vi "DSA AI and AO.vi"() -> ()   [LabVIEW 2014]
doc: "Overview:\nThis VI demonstrates generation and acquisition of a broadband signal to perform measurement of the frequency response of your device.\n\nRequirements:\nLabVIEW Full Development System\nSound and Vibration Toolkit\n\nInstructions:\n1. Connect DUT to DAQmx hardware.\n2. Specify connected output channel and input channel.\n3. Use SVL Measure Propagation Delay (DAQmx) VI to measure device propagation delay [samples].\n4. Run the VI.\n\nDetails:\nThis VI generates and acquires data for an averaged frequency response measurement. This VI performs a continuous acquisition and stops when the averaged measurement is complete. You specify the sampling frequency, block size, and averaging parameters to use for the frequency response measurement. \n\nThe graph outputs display the acquired stimulus and response signals versus time and the magnitude and phase of the frequency response versus frequency."
uses:
  <vilib>/addons/_NISVFA/_Shared subVIs/Controls/svc_Window.ctl
  <vilib>/Utility/error.llb/DialogType.ctl
  <vilib>/DAQmx/create/channels.llb/DAQmx Create Channel (AI-Voltage-Basic).vi
  <vilib>/DAQmx/configure/timing.llb/DAQmx Timing (Sample Clock).vi
  <vilib>/DAQmx/create/channels.llb/DAQmx Create Channel (AO-Voltage-Basic).vi
  <vilib>/DAQmx/configure/trigger.llb/DAQmx Start Trigger (Digital Edge).vi
  <vilib>/DAQmx/write.llb/DAQmx Write (Analog 2D DBL NChan NSamp).vi
  <vilib>/DAQmx/read.llb/DAQmx Read (Analog 1D Wfm NChan NSamp).vi
  <vilib>/addons/_NISVFA/_Baseband FFT/SVFA Power Spectrum (1 Ch).vi
  <vilib>/Analysis/NI_AALBase.lvlib
  <resource>/objmgr/daqmx.rc
  <vilib>/measure/NI_MABase.lvlib
panel:
  out "DC 2":dbl min=0.0 max=1.0 step=0.001 format="%.3f"
  out "DC 1":dbl min=0.0 max=1.0 step=0.001 format="%.3f"
  out "RMS 2":dbl min=0.0 max=1.0 step=0.001 format="%.3f"
  out "RMS 1":dbl min=0.0 max=1.0 step=0.001 format="%.3f"
  in  "stop":bool
  in  "Tab Control":enum32{"Time Record", "Power Spectum"}(tab)
  out "time record 2":waveform(dbl)[](graph)
  in  "sampling rate [Hz]":dbl=51200.0 format="%.2f"
  out "actual update rate":dbl=51200.0 format="%.2f"
  in  "excitation":T1(ring)=enum."Sine"
  in  "output physical channel":tag="PXI2Slot4/ao0:1"
  in  "input channel (stimulus)":tag="PXI2Slot4/ai0"
  in  "propagation delay [samples]":i32=1 min=1 step=1
  in  "amplitude":dbl=0.1 min=0.0 max=2.0 step=0.001 format="%.3f"
  in  "input channel (response)":tag="PXI2Slot4/ai1"
  in  "frequency":dbl=150.0 min=0.0 max=20000.0 step=0.1 format="%.1f"
  out "mag 2":cluster{"f0":dbl, "df":dbl, "magnitude":dbl[]}(graph)={"f0"=0.0, "df"=20.00000050524251, "magnitude"=[]}
  out "mag":cluster{"f0":dbl, "df":dbl, "magnitude":dbl[]}(graph)={"f0"=0.0, "df"=20.00000050524251, "magnitude"=[]}
  in  "block size":i32=16384 min=128
  in  "averaging parameters":T2={"averaging mode"=enum."RMS averaging", "weighting mode"=enum."Exponential", "number of averages"=10, "linear mode"=enum."One shot"} {"number of averages" min=1 step=1}
  in  "restart averaging":bool
  out "averages completed":dbl
  in  "window":T3=1 items=["None"=0, "Hanning"=1, "Hamming"=2, "Blackman-Harris"=3, "Exact Blackman"=4, "Blackman"=5, "Flat Top"=6, "4 Term B-Harris "=7, "7 Term B-Harris"=8, "Low Sidelobe"=9, "Force"=64, "Exponential"=65, "Blackman Nuttall"=11, "Triangle"=30, "Bartlett-Hanning"=31, "Bohman"=32, "Parzen"=33, "Welch"=34, "Kaiser"=60, "Dolph-Chebyshev"=61, "Gaussian"=62]
  in  "dB On":bool=TRUE
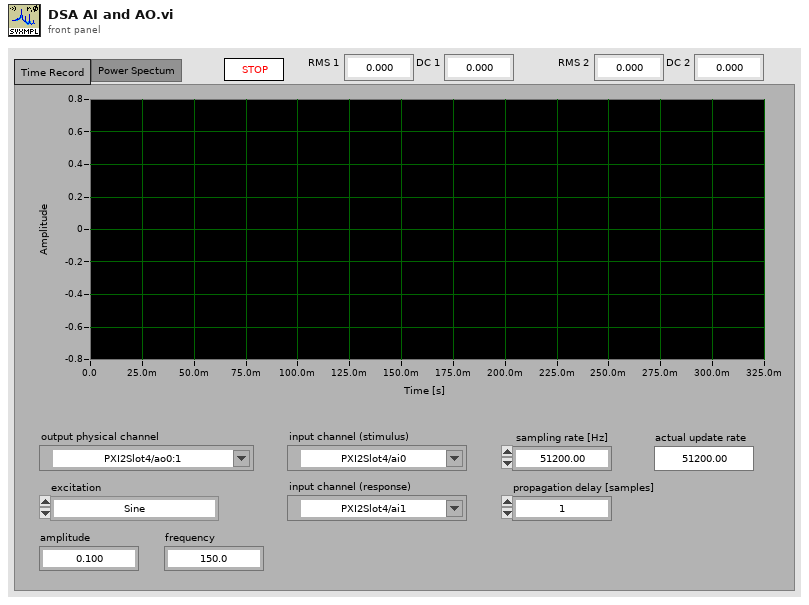
[diagram p1: front panel]
types:
  T1 = enum16{"uniform white noise", "Gaussian white noise", "periodic random noise", "Chirp", "Sine"}
  T2 = cluster{"averaging mode":enum16{"No averaging", "Vector averaging", "RMS averaging", "Peak hold"}, "weighting mode":enum16{"Linear", "Exponential"}, "number of averages":u32, "linear mode":enum16{"One shot", "Auto restart"}}
  T3 = typedef "svc_Window.ctl" = u32
  T4 = cluster{"coupling":i32, "enable IEPE excitation":bool, "IEPE current [mA]":dbl}
  T5 = typedef "DialogType.ctl" = u16
  T6 = cluster{"actual sample rate":dbl, "block size":i32}
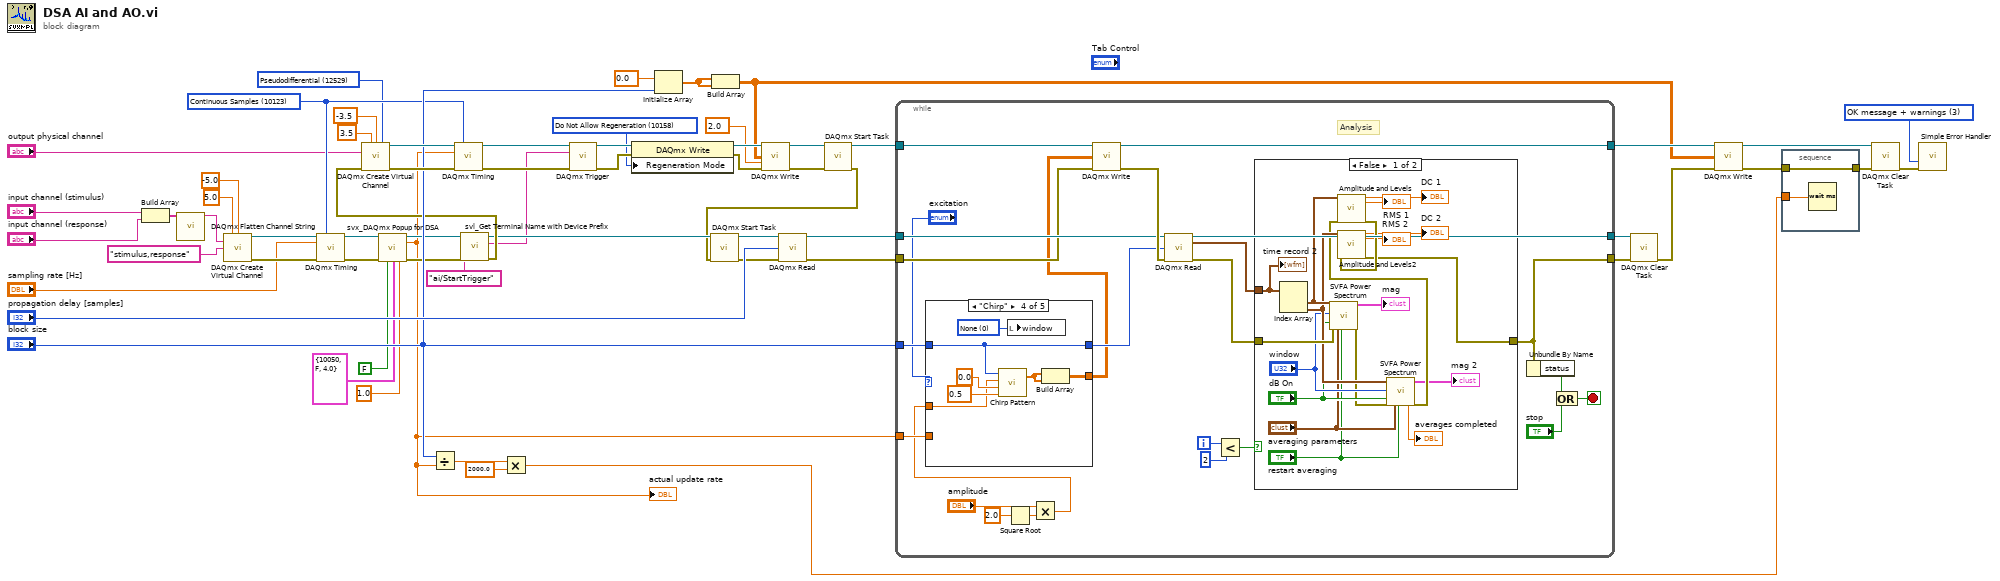
[diagram p0: block diagram]
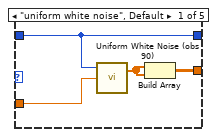
[diagram p2: hidden frame]
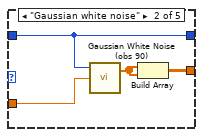
[diagram p3: hidden frame]
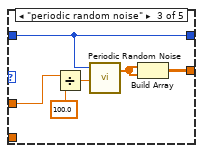
[diagram p4: hidden frame]
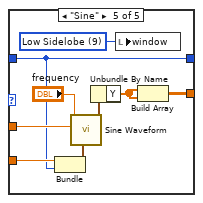
[diagram p5: hidden frame]
diagram:
  w3 = 12529 items=["Default"=-1, "RSE"=10083, "Differential"=10106, "Pseudodifferential"=12529] ("output terminal configuration")
  w30 = T5 3 items=["no dialog", "OK message", "continue or stop message", "OK message + warnings", "continue/stop + warnings"] ("type of dialog (OK msg:1)")
  w51 = 10158 items=["Allow Regeneration"=10097, "Do Not Allow Regeneration"=10158] ("RegenMode")
  w17 = 10123 items=["Finite Samples"=10178, "Continuous Samples"=10123] ("sample mode")
  n1 = Build Array("input channel (stimulus)", "input channel (response)") -> (w12:tag[])
  n2 = call <vilib>:"DAQmx Flatten Channel String.vi"("names in"=w12) -> ("names out"=w9:string)  [unwired: 13 in, 1 out]
  n3 = call-poly <vilib>:"DAQmx Create Virtual Channel.vi"("maximum value"=5.0, "minimum value"=-5.0, "physical channels"=w9, "name to assign"="stimulus,response") -> ("task out"=w29:refnum<k21>, "error out"=w28:errorcluster)  [unwired: 10 in]
  n4 = call-poly <vilib>:"DAQmx Timing.vi"("task/channels in"=w29, "sample mode"=w17, "rate"="sampling rate [Hz]", "error in"=w28) -> ("task out"=w14:refnum<k21>, "error out"=w13:errorcluster)  [unwired: 10 in]
  n5 = call <vilib>:"svx_DAQmx Popup for DSA.vi"("task in"=w14, "error in (no error)"=w13, "interactive configuration dialog"=FALSE, "DSA channel settings"=T4 {"coupling"=10050, "enable IEPE excitation"=FALSE, "IEPE current [mA]"=4.0}, "time to settle [s]"=1.0) -> ("task out"=w24:refnum<k21>, "actual sample rate"=w7:dbl, "error out"=w23:errorcluster)  [unwired: 8 in]
  "actual update rate" <- w7
  n6 = Divide(x="block size", y=w7) -> (x/y=w36:dbl)
  n7 = call <vilib>:"svl_Get Terminal Name with Device Prefix.vi"("error in (no error)"=w23, "local terminal name"="ai/StartTrigger", "task/channels in"=w24) -> ("error out"=w27:errorcluster, "terminal name with device prefix"=w16:tag, "task out"=w26:refnum<k21>)  [unwired: 6 in]
  n8 = call-poly <vilib>:"DAQmx Create Virtual Channel.vi"("maximum value"=3.5, "minimum value"=-3.5, "output terminal configuration"=w3, "physical channels"="output physical channel", "error in"=w27) -> ("task out"=w61:refnum<k21>, "error out"=w60:errorcluster)  [unwired: 9 in]
  n9 = call-poly <vilib>:"DAQmx Timing.vi"("task/channels in"=w61, "sample mode"=w17, "rate"=w7, "error in"=w60) -> ("task out"=w59:refnum<k21>, "error out"=w58:errorcluster)  [unwired: 10 in]
  n10 = Multiply(x=w36, y=2000.0) -> (x*y=w34:dbl)
  n11 = call-poly <vilib>:"DAQmx Trigger.vi"("task/channels in"=w59, "source"=w16, "error in"=w58) -> ("task out"=w55:refnum<k21>, "error out"=w54:errorcluster)  [unwired: 11 in]
  n12 = property class="DAQmx Write"(reference=w55, error in=w54, "Regeneration Mode"=w51) -> (reference out=w53:refnum<k21>, error out=w52:errorcluster)
  n13 = Initialize Array(0.0 ("element"), "block size") -> (w2:dbl[])
  n14 = Build Array(w2, w2) -> (w1:dbl[][])
  n15 = call-poly <vilib>:"DAQmx Write.vi"("task/channels in"=w53, "data"=w1, "timeout"=2.0 ("Wirite Timeout"), "error in"=w52) -> ("task out"=w57:refnum<k21>, "error out"=w56:errorcluster)  [unwired: 9 in, 1 out]
  n16 = call <vilib>:"DAQmx Start Task.vi"("task/channels in"=w57, "error in"=w56) -> ("task out"=w45:refnum<k21>, "error out"=w25:errorcluster)  [unwired: 12 in]
  n17 = call <vilib>:"DAQmx Start Task.vi"("task/channels in"=w26, "error in"=w25) -> ("task out"=w31:refnum<k21>, "error out"=w32:errorcluster)  [unwired: 12 in]
  n18 = call-poly <vilib>:"DAQmx Read.vi"("task/channels in"=w31, "number of samples per channel"="propagation delay [samples]", "error in"=w32) -> ("task out"=w44:refnum<k21>, "error out"=w43:errorcluster)  [unwired: 10 in, 1 out]
  n19 = while {
    tunnel: "block size" -> [w84]
    tunnel: w43 -> [w73]
    tunnel: [w81] -> w42
    tunnel: [w72] -> w49
    tunnel: [w71] -> w48
    tunnel: w45 -> [w75]
    tunnel: w44 -> [w74]
    tunnel: w7 -> [w69]
    i -> [w86]
    stop <- w82 stop-if-true
    # "Analysis"
    n20 = Square Root(x=2.0 ("y")) -> (sqrt(x)=w66:dbl)
    n21 = Multiply(x="amplitude", y=w66) -> (x*y=w63:dbl)
    n22 = case shown="\"Chirp\"" "excitation" {
      tunnel: [w88 w92 w96 w103 w111] -> w68
      tunnel: w84 -> [w90 w94 w100 w107 w114]
      tunnel: [w90 w94 w100 w107 w114] -> w76
      tunnel: w63 -> [w89 w93 w98 w104 w116]
      tunnel: w69 -> [_ _ _ _ w115]
      frame "uniform white noise", Default {
        n23 = call <vilib>:"Uniform White Noise (obs 90).vi"("amplitude"=w89, "samples"=w90) -> ("uniform white noise"=w87:dbl[])  [unwired: 1 in, 1 out]
        n24 = Build Array(w87, w87) -> (w88:dbl[][])
      }
      frame "Gaussian white noise" {
        n25 = call <vilib>:"Gaussian White Noise (obs 90).vi"("standard deviation"=w93, "samples"=w94) -> ("Gaussian noise pattern"=w91:dbl[])  [unwired: 1 in, 1 out]
        n26 = Build Array(w91, w91) -> (w92:dbl[][])
      }
      frame "periodic random noise" {
        n27 = Divide(x=w98, y=100.0) -> (x/y=w97:dbl)
        n28 = call <vilib>:"Periodic Random Noise.vi"("spectral amplitude"=w97, "samples"=w100) -> ("periodic random noise"=w95:dbl[])  [unwired: 1 in, 1 out]
        n29 = Build Array(w95, w95) -> (w96:dbl[][])
      }
      frame "Chirp" {
        w101 = T3 0 items=["None"=0, "Hanning"=1, "Hamming"=2, "Blackman-Harris"=3, "Exact Blackman"=4, "Blackman"=5, "Flat Top"=6, "4 Term B-Harris "=7, "7 Term B-Harris"=8, "Low Sidelobe"=9, "Force"=64, "Exponential"=65, "Blackman Nuttall"=11, "Triangle"=30, "Bartlett-Hanning"=31, "Bohman"=32, "Parzen"=33, "Welch"=34, "Kaiser"=60, "Dolph-Chebyshev"=61, "Gaussian"=62] ("window")
        n30 = call <vilib>:"Chirp Pattern.vi"("f2"=0.5, "f1"=0.0, "amplitude"=w104, "samples"=w107) -> ("Chirp Pattern"=w102:dbl[])  [unwired: 1 out]
        n31 = local write "window"(w101) -> ()
        n32 = Build Array(w102, w102) -> (w103:dbl[][])
      }
      frame "Sine" {
        w108 = T3 9 items=["None"=0, "Hanning"=1, "Hamming"=2, "Blackman-Harris"=3, "Exact Blackman"=4, "Blackman"=5, "Flat Top"=6, "4 Term B-Harris "=7, "7 Term B-Harris"=8, "Low Sidelobe"=9, "Force"=64, "Exponential"=65, "Blackman Nuttall"=11, "Triangle"=30, "Bartlett-Hanning"=31, "Bohman"=32, "Parzen"=33, "Welch"=34, "Kaiser"=60, "Dolph-Chebyshev"=61, "Gaussian"=62] ("window")
        n33 = Bundle("actual sample rate"=w115, "block size"=w114) -> (w113:T6)  [unwired: 1 in]
        n34 = call <vilib>:"Sine Waveform.vi"("sampling info"=w113, "amplitude"=w116, "frequency"="frequency") -> ("signal out"=w112:waveform(dbl))  [unwired: 7 in, 1 out]
        n35 = Unbundle By Name(w112) -> ("Y"=w110:dbl[])
        n36 = local write "window"(w108) -> ()
        n37 = Build Array(w110, w110) -> (w111:dbl[][])
      }
    }
    n38 = call-poly <vilib>:"DAQmx Write.vi"("task/channels in"=w75, "data"=w68, "error in"=w73) -> ("task out"=w72:refnum<k21>, "error out"=w79:errorcluster)  [unwired: 10 in, 1 out]
    n39 = call-poly <vilib>:"DAQmx Read.vi"("task/channels in"=w74, "number of samples per channel"=w76, "error in"=w79) -> ("task out"=w71:refnum<k21>, "data"=w77:waveform(dbl)[], "error out"=w78:errorcluster)  [unwired: 10 in]
    n40 = Less?(x=w86, y=2) -> (x < y?=w85:bool)
    n41 = case shown="False" w85 {
      tunnel: w78 -> [w135 w136]
      tunnel: w77 -> [w133 _]
      tunnel: [w130 w136] -> w81
      frame False {
        n42 = Index Array(array=w133) -> (element #1=w132:waveform(dbl), element #2=w125:waveform(dbl))  [unwired: 2 in]
        n43 = call-poly <vilib>:"SVFA Power Spectrum.vi"("scaled signal [EU]"=w132, "window"="window", "dB On (T)"="dB On", "error in (no error)"=w135, "averaging parameters"="averaging parameters", "restart averaging (F)"="restart averaging") -> ("power spectrum [dB EU]"=→"mag":cluster{"f0":dbl, "df":dbl, "magnitude":dbl[]}, "error out"=w122:errorcluster)  [unwired: 8 in, 4 out]
        n44 = call-poly <vilib>:"SVFA Power Spectrum.vi"("scaled signal [EU]"=w125, "window"="window", "dB On (T)"="dB On", "error in (no error)"=w122, "averaging parameters"="averaging parameters", "restart averaging (F)"="restart averaging") -> ("averages completed"=→"averages completed":dbl, "power spectrum [dB EU]"=→"mag 2":cluster{"f0":dbl, "df":dbl, "magnitude":dbl[]}, "error out"=w121:errorcluster)  [unwired: 8 in, 3 out]
        n45 = call "Amplitude and Levels"("input signal"=w132, "error in"=w121) -> ("dc"=→"DC 1":dbl, "rms"=→"RMS 1":dbl, "error out"=w131:errorcluster)  [unwired: 15 in]
        n46 = call "Amplitude and Levels2"("input signal"=w125, "error in"=w131) -> ("dc"=→"DC 2":dbl, "rms"=→"RMS 2":dbl, "error out"=w130:errorcluster)  [unwired: 15 in]
        "time record 2" <- w133
      }
      frame True {
        # "discard first buffer (\"0\")"
      }
    }
    n47 = Unbundle By Name(w81) -> ("status"=w83:bool)
    n48 = Compound Arithmetic op=OR(w83, "stop") -> (w82:bool)
  }
  n49 = call <vilib>:"DAQmx Clear Task.vi"("task in"=w48, "error in"=w42) -> ("error out"=w41:errorcluster)  [unwired: 13 in]
  n50 = call-poly <vilib>:"DAQmx Write.vi"("task/channels in"=w49, "data"=w1, "error in"=w41) -> ("task out"=w40:refnum<k21>, "error out"=w39:errorcluster)  [unwired: 10 in, 1 out]
  n51 = stacked-sequence {
    tunnel: w39 -> [w138]
    tunnel: [w138] -> w38
    tunnel: w34 -> [w137]
    frame #0 {
      n52 = Wait (ms)(milliseconds to wait=w137) -> ()  [unwired: 1 out]
    }
  }
  n53 = call <vilib>:"DAQmx Clear Task.vi"("task in"=w40, "error in"=w38) -> ("error out"=w50:errorcluster)  [unwired: 13 in]
  n54 = call <vilib>:"Simple Error Handler.vi"("type of dialog (OK msg:1)"=w30, "error in (no error)"=w50) -> ()  [unwired: 3 in, 5 out]
